vi "Accelerometer.vi"   [LabVIEW 2016]
uses:
  <vilib>/rvi/eio/common/nirviEmuTemplateMethod_errors.vi
  <vilib>/eio/EIONode/EIONode.xnode
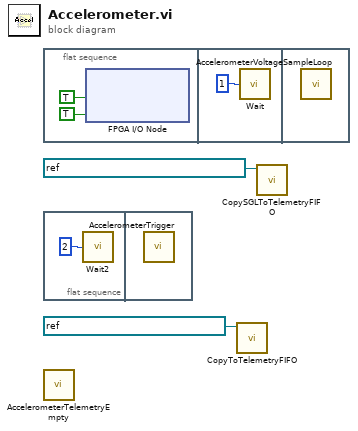
[diagram p0: block diagram]
diagram:
  n1 = flat-sequence {
    frame #0 {
      n2 = xnode "FPGA I/O Node"("Mod1/Start"=TRUE, "Mod2/Start"=TRUE) -> ()  [unwired: 2 in, 2 out]
    }
    frame #1 {
      n3 = call "Wait"("Count(mSec)"=u8 1) -> ()  [unwired: 1 out]
    }
    frame #2 {
      n4 = call "AccelerometerVoltageSampleLoop.vi"() -> ()  [unwired: 12 in]
    }
  }
  n5 = flat-sequence {
    frame #0 {
      n6 = call "Wait2"("Count(mSec)"=u8 2) -> ()  [unwired: 1 out]
    }
    frame #1 {
      n7 = call "AccelerometerTrigger.vi"() -> ()  [unwired: 12 in]
    }
  }
  n8 = call "AccelerometerTelemetryEmpty.vi"() -> ()  [unwired: 12 in]
  n9 = call "CopyToTelemetryFIFO.vi"("SourceFIFO"=refnum<k21> "AccelerometerTelemetryFIFO") -> ()  [unwired: 11 in]
  n10 = call "CopySGLToTelemetryFIFO.vi"("SourceFIFO"=refnum<k21> "AccelerometerTelemetrySGLFIFO") -> ()  [unwired: 11 in]
